vi "%s (Request & Reply).vi"(7 "Additional Reply Message Queues (Default 0)":i32, 8 "error in (no error)":errorcluster, 11 "API-Reference in":refnum<data-value>) -> (0 "error out":errorcluster, 3 "API-Reference out":refnum<data-value>)   [LabVIEW 2018, in "Scripting.lvlib" / "Actor.lvclass"]
uses:
  Actor.lvclass
  Request-Enqueuers.ctl
  Did Stop.ctl
  API-Data.ctl
  Front-Panel State.ctl
  Did Initialize.ctl
  Broadcast Enqueuers.ctl
  All-Enqueuers.ctl
  State.ctl
  Get State.ctl
  Stop.ctl
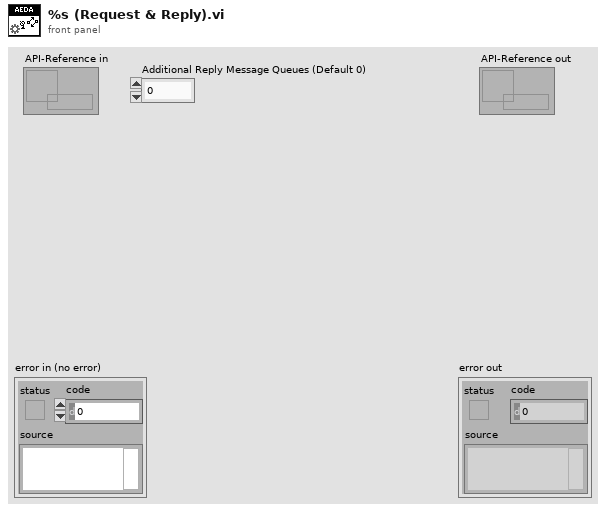
[diagram p1: front panel]
types:
  T1 = typedef "Scripting.lvlib/Actor.lvclass/API-Data.ctl" = cluster{"Launch":refnum<notifier>, "Did Stop Message":refnum<event-registration>, "Did Stop Enqueuer":refnum<user-event>, "Enqueuers":T2}
  T2 = typedef "Scripting.lvlib/Actor.lvclass/All-Enqueuers.ctl" = cluster{"Broadcasts":T3, "Requests":T4}
  T3 = typedef "Scripting.lvlib/Actor.lvclass/Broadcast Enqueuers.ctl" = cluster{"Did Initialize":refnum<user-event>}
  T4 = typedef "Scripting.lvlib/Actor.lvclass/Request-Enqueuers.ctl" = cluster{"Get State":refnum<user-event>, "Stop":refnum<user-event>}
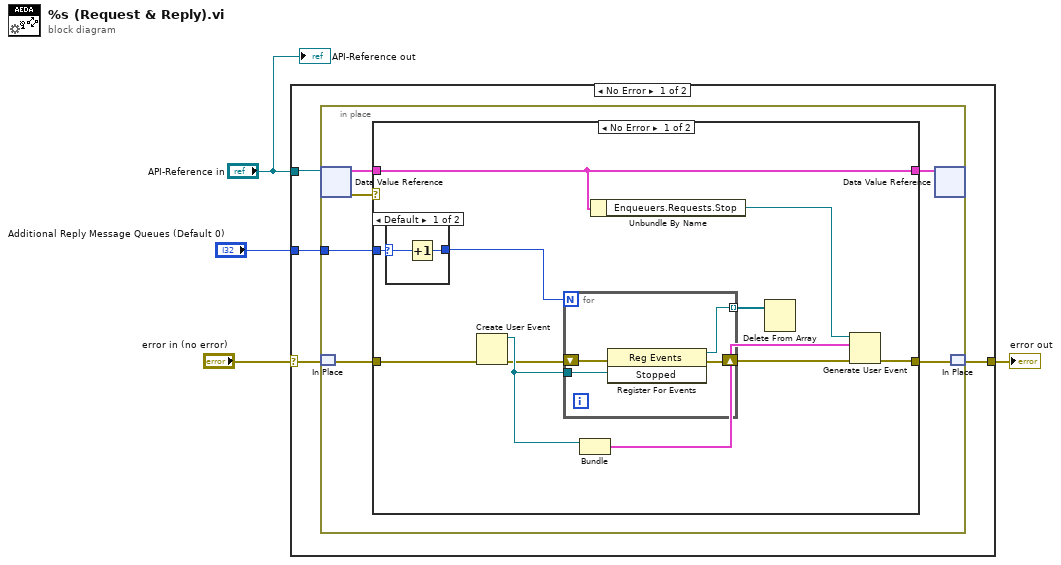
[diagram p0: block diagram]
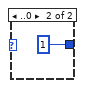
[diagram p2: hidden frame]
diagram:
  n1 = case shown="No Error" "error in (no error)" {
    selector: "error in (no error)" -> [w8 w35]
    tunnel: [w7 w35] -> w3
    tunnel: "API-Reference in" -> [w6 _]
    tunnel: "Additional Reply Message Queues (Default 0)" -> [w5 _]
    frame No Error {
      n2 = in-place {
        in-place-border: w5 -> [w9]
        n3 = in-place-dvr #1(w6) -> (w13:T1, w14:errorcluster)
        n4 = in-place-match #2(w8) -> (w11:errorcluster)
        n5 = case shown="No Error" w14 {
          selector: w14 -> [_ w34]
          tunnel: w13 -> [w25 w33]
          tunnel: [w25 w33] -> w12
          tunnel: w11 -> [w24 _]
          tunnel: [w22 w34] -> w10
          tunnel: w9 -> [w19 _]
          frame No Error {
            n6 = case shown="Default" w19 {
              selector: w19 -> [w27 _]
              tunnel: [w26 1] -> w18
              frame Default {
                n7 = Increment(x=w27) -> (x+1=w26:i32)
              }
              frame ..0 {
              }
            }
            n8 = Create User Event(error in=w24) -> (user event=w20:refnum<user-event>, error out=w17:errorcluster)  [unwired: 1 in]
            n9 = for {
              N: w18 -> [_]
              shift-right: [w31] -> w23
              shift-left: w17 -> [w32]
              tunnel: [w30] -> w16 mode=indexing
              tunnel: w20 -> [w29]
              n10 = register-events(error in=w32, w29) -> (reference out=w30:refnum<event-registration>, error out=w31:errorcluster)  [unwired: 1 in]
            }
            n11 = Bundle("Stopped"=w20) -> (w15:cluster{"Stopped":refnum<user-event>, void})  [unwired: 2 in]
            n12 = Unbundle By Name(w25) -> ("Enqueuers.Requests.Stop"=w21:refnum<user-event>)
            n13 = Delete From Array(array=w16) -> ()  [unwired: 2 in, 2 out]
            n14 = Generate User Event(user event=w21, event data cluster=w15, error in=w23) -> (error out=w22:errorcluster)  [unwired: 1 in, 1 out]
          }
          frame Error {
          }
        }
        n15 = in-place-dvr #1(w12) -> ()  [unwired: 2 out]
        n16 = in-place-match #2(w10) -> (w7:errorcluster)
      }
    }
    frame Error {
    }
  }
  "error out" <- w3
  "API-Reference out" <- "API-Reference in"
